vi "score.vi"(8 "error in (no error)":errorcluster caption="entrée d'erreur (pas d'erreur)", 11 "MultiTaskLasso.lvclass 2":refnum<class "MultiTaskLasso.lvclass">) -> (0 "error out":errorcluster caption="sortie d'erreur", 2 "score":dbl, 3 "MultiTaskLasso.lvclass":refnum<class "MultiTaskLasso.lvclass">)   [LabVIEW 2020, in "MultiTaskLasso.lvclass"]
doc: "Return the coefficient of determination :math:`R^2` of the\n prediction.\n\n The coefficient :math:`R^2` is defined as :math:`(1 - \\frac{u}{v})`,\n where :math:`u` is the residual sum of squares ``((y_true - y_pred)\n ** 2).sum()`` and :math:`v` is the total sum of squares ``((y_true -\n y_true.mean()) ** 2).sum()``. The best possible score is 1.0 and it\n can be negative (because the model can be arbitrarily worse). A\n constant model that always predicts the expected value of `y`,\n disregarding the input features, would get a :math:`R^2` score of\n 0.0."
uses:
  MultiTaskLasso.lvclass
  C:/Users/cipop/TDF Dropbox/2_Technologies de France/1 - Services et Etudes/PLAIY/2 - DEV/PLAIYLAB/code/Python/Python.lvclass
  C:/Users/cipop/TDF Dropbox/2_Technologies de France/1 - Services et Etudes/PLAIY/2 - DEV/PLAIYLAB/code/Model/Model.lvclass
  MultiTaskLasso.lvclass/MultiTaskLasso.ctl
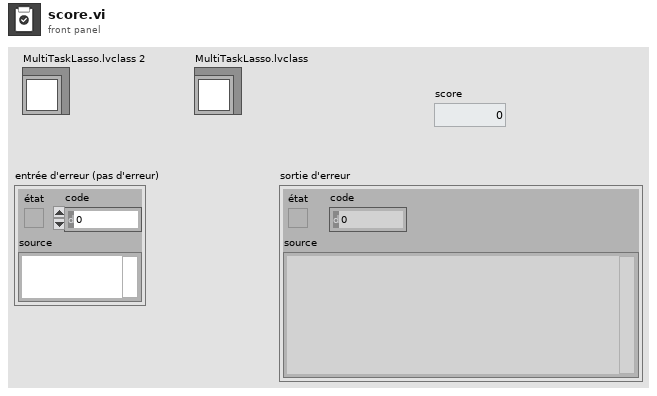
[diagram p1: front panel]
types:
  T1 = typedef "data.ctl" = cluster{"name":string, "X":dbl[][]}
  T2 = typedef "multi_task_lasso_data.ctl" = cluster{"y":dbl[][], "sample_weight":dbl[]}
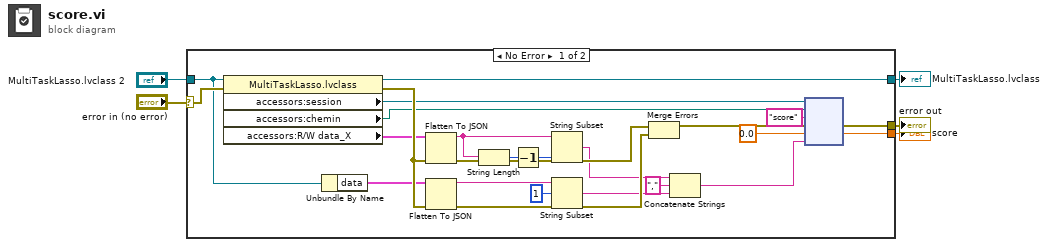
[diagram p0: block diagram]
diagram:
  n1 = case shown="No Error" "error in (no error)" {
    selector: "error in (no error)" -> [w27 w31]
    tunnel: [w28 w31] -> w4
    tunnel: [w10 w30] -> w2
    tunnel: "MultiTaskLasso.lvclass 2" -> [w9 w30]
    tunnel: [w6 _] -> w1
    frame No Error {
      n2 = property class="MultiTaskLasso.lvclass"(reference=w9, error in=w27) -> (reference out=w10:refnum<class "MultiTaskLasso.lvclass">, error out=w23:errorcluster, "accessors:session"=w13:refnum<k35>, "accessors:chemin"=w12:path, "accessors:R/W data_X"=w14:T1)
      n3 = Unbundle By Name(w9) -> ("data"=w8:T2)
      n4 = Flatten To JSON(anything=w14, error in (no error)=w23) -> (JSON string=w24:string, 11:w19:errorcluster)  [unwired: 1 in]
      n5 = Flatten To JSON(anything=w8, error in (no error)=w23) -> (JSON string=w21:string, 11:w20:errorcluster)  [unwired: 1 in]
      n6 = String Length(string=w24) -> (length=w26:i32)
      n7 = Decrement(x=w26) -> (x-1=w25:i32)
      n8 = String Subset(string=w24, length (rest)=w25) -> (substring=w17:string)  [unwired: 1 in]
      n9 = String Subset(string=w21, offset (0)=1) -> (substring=w16:string)  [unwired: 1 in]
      n10 = Merge Errors(w19, w20) -> (w11:errorcluster)
      n11 = Concatenate Strings(w17, "," ("string"), w16) -> (w15:string)
      n12 = node(w13, w12, "score" ("nom de la fonction"), w11, 0.0 ("score"), w15) -> (w28:errorcluster, w6:dbl)  [unwired: 1 in, 3 out]
    }
    frame Error {
    }
  }
  "error out" <- w4
  "MultiTaskLasso.lvclass" <- w2
  "score" <- w1
